vi "Open Utility Motors.vi"(9 "CAN IDs":u8[](array[numeric])=[0, 0, 0, 0, 0, 0, 0]) -> ()   [LabVIEW 2018]
uses:
  <vilib>/Rock Robotics/SystemInterfaces/DIO/FPGA_DIOChannel.ctl
  <vilib>/Rock Robotics/WPI/ThirdParty/Phoenix-LabVIEW/Motor Controller/Controls/CTRE_Phoenix_MotorControl_NeutralMode.ctl
  <vilib>/Rock Robotics/WPI/Switch/WPI_SwitchOpenLimit.vi
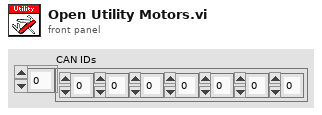
[diagram p1: front panel]
types:
  T1 = typedef "CTRE_Phoenix_MotorControl_NeutralMode.ctl" = enum8{"EEPROMSetting", "Override to Coast", "Override to Brake"}
  T2 = typedef "FPGA_DIOChannel.ctl" = enum8{"DIO 0", "DIO 1", "DIO 2", "DIO 3", "DIO 4", "DIO 5", "DIO 6", "DIO 7", "DIO 8", "DIO 9", "DIO MXP 0", "DIO MXP 1", "DIO MXP 2", "DIO MXP 3", "DIO MXP 4", "DIO MXP 5", "DIO MXP 6", "DIO MXP 7", "DIO MXP 8", "DIO MXP 9", "DIO MXP 10", "DIO MXP 11", "DIO MXP 12", "DIO MXP 13", "DIO MXP 14", "DIO MXP 15", "SPI Port CS1", "SPI Port CS2", "SPI Port CS3", "SPI Port MISO", "SPI Port MOSI", "Invalid"}
  T3 = typedef "WPI_MotorControlDeviceRef.ctl" = cluster{"DeviceStatus":errorcluster, "Type":T4, "PWM":cluster{"PWM Channel":T5, "DeadBand":T6}, "CAN":cluster{"Device Number":u8, "SetOutput VI Ref":variant, "GetOutput VI Ref":variant, "Enable VI Ref":variant, "Disable VI Ref":variant, "Data":variant}, "Invert":bool, "DIO PWM":cluster{"PWM \"Enable\" Channel":T5, "DIOChannel":T2, "PWM Rate":dbl}}
  T4 = typedef "WPI_MotorControlType.ctl" = enum16{"PWM", "CAN", "DIO PWM"}
  T5 = typedef "FPGA_DIOPWMChannel.ctl" = enum8{"PWM 0", "PWM 1", "PWM 2", "PWM 3", "PWM 4", "PWM 5", "PWM 6", "PWM 7", "PWM 8", "PWM 9", "PWM MXP 0", "PWM MXP 1", "PWM MXP 2", "PWM MXP 3", "PWM MXP 4", "PWM MXP 5", "PWM MXP 6", "PWM MXP 7", "PWM MXP 8", "PWM MXP 9", "Invalid"}
  T6 = typedef "WPI_PWMDeadband.ctl" = cluster{"Name":string, "maxPositivePwm":i32, "minPositivePwm":i32, "centerPwm":i32, "maxNegativePwm":i32, "minNegativePwm":i32, "angularRange":u16}
  T7 = typedef "WPI_SwitchDevRef.ctl" = cluster{"DevStatus":errorcluster, "DIO Channel":T2, "CntIndex":T8, "Normally Closed":bool}
  T8 = typedef "FPGA_CounterCtrSystemIndex.ctl" = enum8{"Ctr 0", "Ctr 1", "Ctr 2", "Ctr 3", "Ctr 4", "Ctr 5", "Ctr 6", "Ctr 7", "Invalid"}
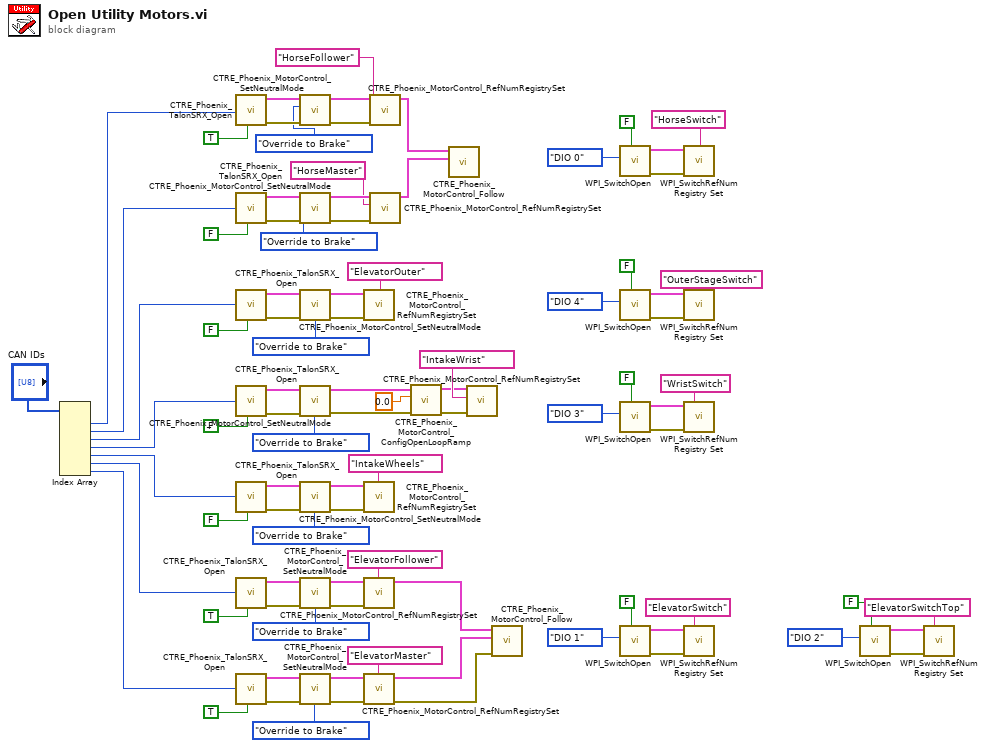
[diagram p0: block diagram]
diagram:
  n1 = Index Array(array="CAN IDs") -> (element #1=w55:u8, element #2=w54:u8, element #3=w53:u8, element #4=w52:u8, element #5=w51:u8, element #6=w50:u8, element #7=w49:u8)  [unwired: 7 in]
  n2 = call <vilib>:"CTRE_Phoenix_TalonSRX_Open.vi"("Invert"=TRUE, "Device Number"=w55) -> ("error out"=w13:errorcluster, "CAN Talon SRX Ref"=w15:T3)  [unwired: 8 in]
  n3 = call <vilib>:"CTRE_Phoenix_TalonSRX_Open.vi"("Invert"=FALSE, "Device Number"=w54) -> ("error out"=w17:errorcluster, "CAN Talon SRX Ref"=w19:T3)  [unwired: 8 in]
  n4 = call <vilib>:"CTRE_Phoenix_TalonSRX_Open.vi"("Invert"=FALSE, "Device Number"=w53) -> ("error out"=w90:errorcluster, "CAN Talon SRX Ref"=w81:T3)  [unwired: 8 in]
  n5 = call <vilib>:"CTRE_Phoenix_TalonSRX_Open.vi"("Invert"=FALSE, "Device Number"=w52) -> ("error out"=w88:errorcluster, "CAN Talon SRX Ref"=w79:T3)  [unwired: 8 in]
  n6 = call <vilib>:"CTRE_Phoenix_TalonSRX_Open.vi"("Invert"=FALSE, "Device Number"=w51) -> ("error out"=w87:errorcluster, "CAN Talon SRX Ref"=w78:T3)  [unwired: 8 in]
  n7 = call <vilib>:"CTRE_Phoenix_TalonSRX_Open.vi"("Invert"=TRUE, "Device Number"=w50) -> ("error out"=w85:errorcluster, "CAN Talon SRX Ref"=w76:T3)  [unwired: 8 in]
  n8 = call <vilib>:"CTRE_Phoenix_TalonSRX_Open.vi"("Invert"=TRUE, "Device Number"=w49) -> ("error out"=w83:errorcluster, "CAN Talon SRX Ref"=w74:T3)  [unwired: 8 in]
  n9 = call <vilib>:"CTRE_Phoenix_MotorControl_SetNeutralMode.vi"("error in (no error)"=w13, "Motor Control Neutral Mode"=CTRE_Phoenix_MotorControl_NeutralMode."Override to Brake", "PhoenixMotorControlDevRef"=w15) -> ("error out"=w12:errorcluster, "PhoenixMotorControlDevRef"=w14:T3)  [unwired: 7 in]
  n10 = call <vilib>:"CTRE_Phoenix_MotorControl_SetNeutralMode.vi"("error in (no error)"=w17, "Motor Control Neutral Mode"=CTRE_Phoenix_MotorControl_NeutralMode."Override to Brake", "PhoenixMotorControlDevRef"=w19) -> ("error out"=w16:errorcluster, "PhoenixMotorControlDevRef"=w18:T3)  [unwired: 7 in]
  n11 = call <vilib>:"CTRE_Phoenix_MotorControl_SetNeutralMode.vi"("error in (no error)"=w90, "Motor Control Neutral Mode"=CTRE_Phoenix_MotorControl_NeutralMode."Override to Brake", "PhoenixMotorControlDevRef"=w81) -> ("error out"=w89:errorcluster, "PhoenixMotorControlDevRef"=w80:T3)  [unwired: 7 in]
  n12 = call <vilib>:"CTRE_Phoenix_MotorControl_SetNeutralMode.vi"("error in (no error)"=w88, "Motor Control Neutral Mode"=CTRE_Phoenix_MotorControl_NeutralMode."Override to Brake", "PhoenixMotorControlDevRef"=w79) -> ("error out"=w5:errorcluster, "PhoenixMotorControlDevRef"=w4:T3)  [unwired: 7 in]
  n13 = call <vilib>:"CTRE_Phoenix_MotorControl_SetNeutralMode.vi"("error in (no error)"=w87, "Motor Control Neutral Mode"=CTRE_Phoenix_MotorControl_NeutralMode."Override to Brake", "PhoenixMotorControlDevRef"=w78) -> ("error out"=w86:errorcluster, "PhoenixMotorControlDevRef"=w77:T3)  [unwired: 7 in]
  n14 = call <vilib>:"CTRE_Phoenix_MotorControl_SetNeutralMode.vi"("error in (no error)"=w85, "Motor Control Neutral Mode"=CTRE_Phoenix_MotorControl_NeutralMode."Override to Brake", "PhoenixMotorControlDevRef"=w76) -> ("error out"=w84:errorcluster, "PhoenixMotorControlDevRef"=w75:T3)  [unwired: 7 in]
  n15 = call <vilib>:"CTRE_Phoenix_MotorControl_SetNeutralMode.vi"("error in (no error)"=w83, "Motor Control Neutral Mode"=CTRE_Phoenix_MotorControl_NeutralMode."Override to Brake", "PhoenixMotorControlDevRef"=w74) -> ("error out"=w82:errorcluster, "PhoenixMotorControlDevRef"=w73:T3)  [unwired: 7 in]
  n16 = call <vilib>:"CTRE_Phoenix_MotorControl_RefNumRegistrySet.vi"("error in (no error)"=w89, "refnum name"="ElevatorOuter", "PhoenixMotorControlDevRef"=w80) -> ()  [unwired: 7 in, 2 out]
  n17 = call <vilib>:"CTRE_Phoenix_MotorControl_RefNumRegistrySet.vi"("error in (no error)"=w86, "refnum name"="IntakeWheels", "PhoenixMotorControlDevRef"=w77) -> ()  [unwired: 7 in, 2 out]
  n18 = call <vilib>:"CTRE_Phoenix_MotorControl_RefNumRegistrySet.vi"("error in (no error)"=w84, "refnum name"="ElevatorFollower", "PhoenixMotorControlDevRef"=w75) -> ("PhoenixMotorControlDevRef"=w47:T3)  [unwired: 7 in, 1 out]
  n19 = call <vilib>:"CTRE_Phoenix_MotorControl_RefNumRegistrySet.vi"("error in (no error)"=w82, "refnum name"="ElevatorMaster", "PhoenixMotorControlDevRef"=w73) -> ("error out"=w45:errorcluster, "PhoenixMotorControlDevRef"=w46:T3)  [unwired: 7 in]
  n20 = call <vilib>:"CTRE_Phoenix_MotorControl_RefNumRegistrySet.vi"("error in (no error)"=w12, "refnum name"="HorseFollower", "PhoenixMotorControlDevRef"=w14) -> ("PhoenixMotorControlDevRef"=w11:T3)  [unwired: 7 in, 1 out]
  n21 = call <vilib>:"CTRE_Phoenix_MotorControl_RefNumRegistrySet.vi"("error in (no error)"=w16, "refnum name"="HorseMaster", "PhoenixMotorControlDevRef"=w18) -> ("PhoenixMotorControlDevRef"=w10:T3)  [unwired: 7 in, 1 out]
  n22 = call <vilib>:"CTRE_Phoenix_MotorControl_ConfigOpenLoopRamp.vi"("error in (no error)"=w5, "secondsFromNeutralToFull"=0.0, "PhoenixMotorControlDevRef"=w4) -> ("error out"=w3:errorcluster, "PhoenixMotorControlDevRef"=w2:T3)  [unwired: 7 in]
  n23 = call <vilib>:"CTRE_Phoenix_MotorControl_Follow.vi"("Master Controller to Follow"=w10, "PhoenixMotorControlDevRef"=w11) -> ()  [unwired: 8 in, 2 out]
  n24 = call <vilib>:"CTRE_Phoenix_MotorControl_RefNumRegistrySet.vi"("error in (no error)"=w3, "refnum name"="IntakeWrist", "PhoenixMotorControlDevRef"=w2) -> ()  [unwired: 7 in, 2 out]
  n25 = call <vilib>:"CTRE_Phoenix_MotorControl_Follow.vi"("error in (no error)"=w45, "Master Controller to Follow"=w46, "PhoenixMotorControlDevRef"=w47) -> ()  [unwired: 7 in, 2 out]
  n26 = call-poly <vilib>:"WPI_SwitchOpen.vi"("Normally Closed"=FALSE, "DIO Channel"=FPGA_DIOChannel."DIO 0") -> ("error out"=w43:errorcluster, "SwitchDevRef"=w44:T7)  [unwired: 8 in]
  n27 = call-poly <vilib>:"WPI_SwitchOpen.vi"("Normally Closed"=FALSE, "DIO Channel"=FPGA_DIOChannel."DIO 4") -> ("error out"=w23:errorcluster, "SwitchDevRef"=w22:T7)  [unwired: 8 in]
  n28 = call-poly <vilib>:"WPI_SwitchOpen.vi"("Normally Closed"=FALSE, "DIO Channel"=FPGA_DIOChannel."DIO 3") -> ("error out"=w26:errorcluster, "SwitchDevRef"=w27:T7)  [unwired: 8 in]
  n29 = call-poly <vilib>:"WPI_SwitchOpen.vi"("Normally Closed"=FALSE, "DIO Channel"=FPGA_DIOChannel."DIO 1") -> ("error out"=w40:errorcluster, "SwitchDevRef"=w39:T7)  [unwired: 8 in]
  n30 = call <vilib>:"WPI_SwitchRefNum Registry Set.vi"("error in (no error)"=w43, "refnum name"="HorseSwitch", "SwitchDevRef"=w44) -> ()  [unwired: 7 in, 2 out]
  n31 = call <vilib>:"WPI_SwitchRefNum Registry Set.vi"("error in (no error)"=w23, "refnum name"="OuterStageSwitch", "SwitchDevRef"=w22) -> ()  [unwired: 7 in, 2 out]
  n32 = call <vilib>:"WPI_SwitchRefNum Registry Set.vi"("error in (no error)"=w26, "refnum name"="WristSwitch", "SwitchDevRef"=w27) -> ()  [unwired: 7 in, 2 out]
  n33 = call <vilib>:"WPI_SwitchRefNum Registry Set.vi"("error in (no error)"=w40, "refnum name"="ElevatorSwitch", "SwitchDevRef"=w39) -> ()  [unwired: 7 in, 2 out]
  n34 = call-poly <vilib>:"WPI_SwitchOpen.vi"("Normally Closed"=FALSE, "DIO Channel"=FPGA_DIOChannel."DIO 2") -> ("error out"=w31:errorcluster, "SwitchDevRef"=w32:T7)  [unwired: 8 in]
  n35 = call <vilib>:"WPI_SwitchRefNum Registry Set.vi"("error in (no error)"=w31, "refnum name"="ElevatorSwitchTop", "SwitchDevRef"=w32) -> ()  [unwired: 7 in, 2 out]
